vi "Bioreactor.vi"(2 "Timer":bool=TRUE, 4 "ДМ2":dbl, 5 "УЗ5":dbl) -> (0 "Error output":bool=TRUE, 1 "Насос 3":bool=TRUE)   [LabVIEW 2019]
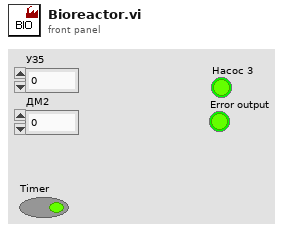
[diagram p1: front panel]
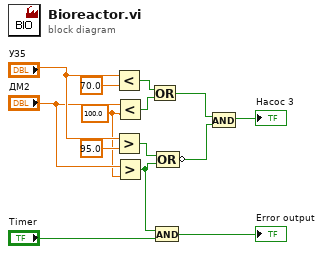
[diagram p0: block diagram]
diagram:
  w5 = 100.0 ("y")
  n1 = Less?(x="УЗ5", y=70.0) -> (x < y?=w13:bool)
  n2 = Greater?(x="УЗ5", y=95.0) -> (0:w10:bool)
  n3 = Less?(x="ДМ2", y=w5) -> (x < y?=w1:bool)
  n4 = Greater?(x="ДМ2", y=w5) -> (0:w4:bool)
  n5 = Or(x=w13, y=w1) -> (x .or. y?=w9:bool)
  n6 = And(x=w4, y="Timer") -> (x .and. y?=→"Error output":bool)
  n7 = Compound Arithmetic op=OR(w10, w4) -> (invert w8:bool)
  n8 = And(x=w9, y=w8) -> (x .and. y?=→"Насос 3":bool)
